vi "XML Reader Start Section.vi"(6 "Default Attribute Values":variant[](array[variant]), 7 "Attribute Names":string[](array[string]), 8 "error in":errorcluster, 10 "Element Name":string, 11 "XML Reader In":T1) -> (0 "error out":errorcluster, 1 "Attribute Values":variant[](array[variant]), 2 "Found?":bool, 3 "XML Reader Out":T1)   [LabVIEW 2018, in "Pathloss XML Reader.lvlib"]
uses:
  Pathloss XML Reader.lvlib
  Controls/XML Reader Data Ref.ctl
  Controls/XML Reader Data.ctl
  <vilib>/Utility/VariantDataType/VariantType.lvlib
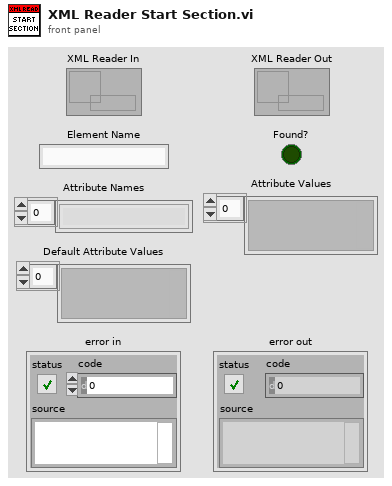
[diagram p1: front panel]
types:
  T1 = typedef "Pathloss XML Reader.lvlib/XML Reader Data Ref.ctl" = refnum<data-value>
  T2 = typedef "Pathloss XML Reader.lvlib/XML Reader Data.ctl" = cluster{"Remaining XML":string, "Section Name Stack":string[], "Section Stack":string[]}
  T3 = typedef "VariantType.lvlib/Type.ctl" = enum8{"Invalid Type", "Void", "I8", "I16", "I32", "I64", "U8", "U16", "U32", "U64", "Single Float", "Double Float", "Extended Float", "Single Complex", "Double Complex", "Extended Complex", "Enum U8", "Enum U16", "Enum U32", "Enum U64", "Single Float With Unit", "Double Float With Unit", "Extended Float With Unit", "Single Complex with Unit", "Double Complex with Unit", "Extended Complex with Unit", "Boolean", "String", "Path", "Picture", "Tag", "Array", "Cluster", "Variant", "LV Variant", "Waveform", "Timestamp", "Digital Waveform", "Digital Data", "ExpressData", "Refnum", "External Data", "VI", "Poly VI", "LabVIEW Class Instance", "Fixed Point"}
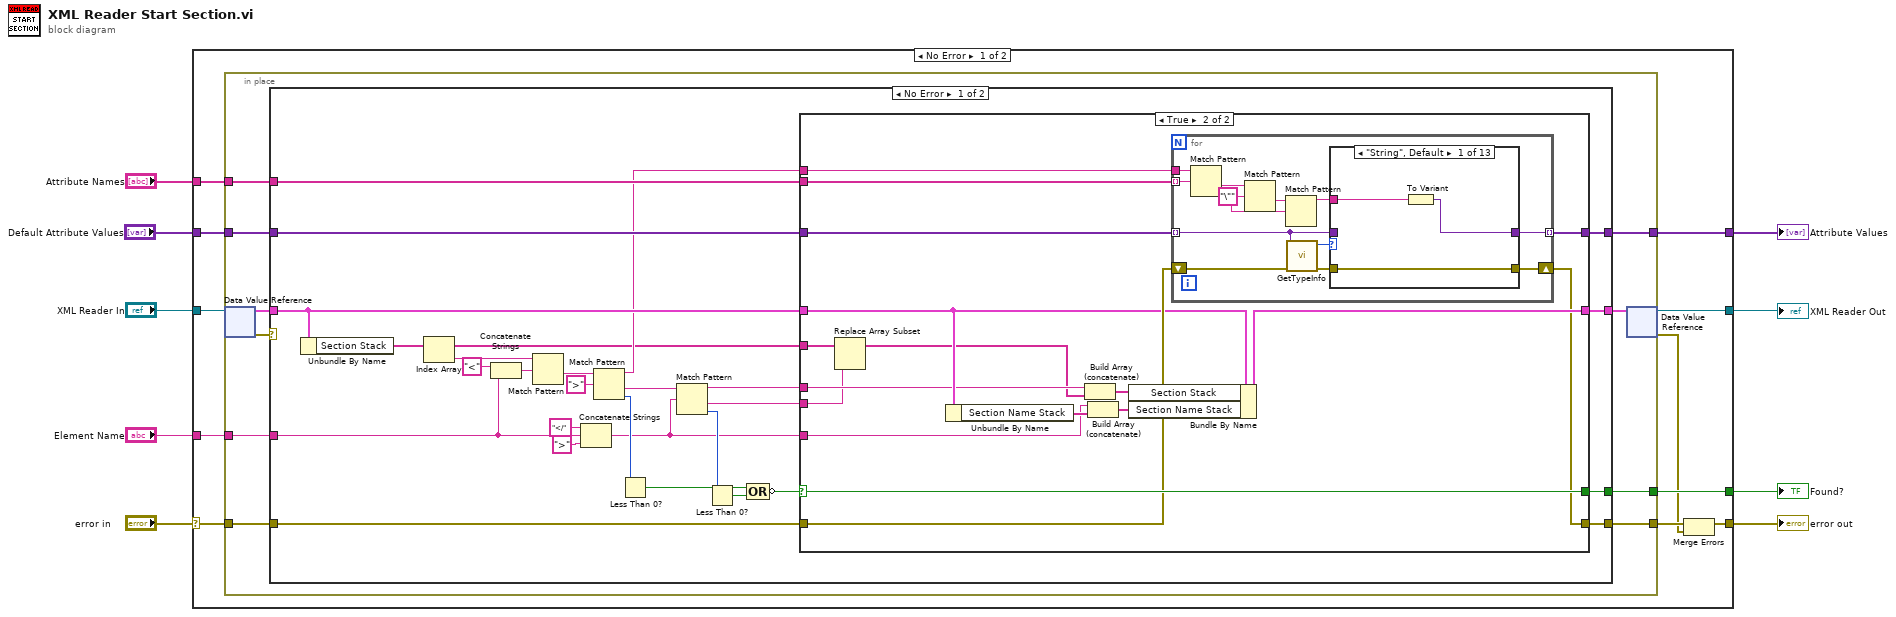
[diagram p0: block diagram]
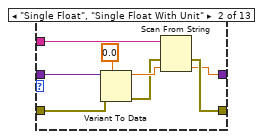
[diagram p3: hidden frame]
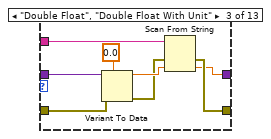
[diagram p4: hidden frame]
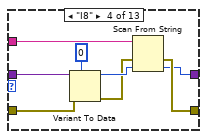
[diagram p5: hidden frame]
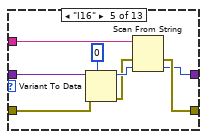
[diagram p6: hidden frame]
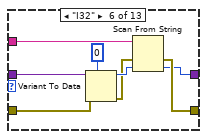
[diagram p7: hidden frame]
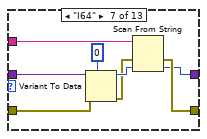
[diagram p8: hidden frame]
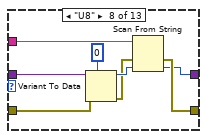
[diagram p9: hidden frame]
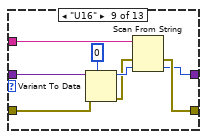
[diagram p10: hidden frame]
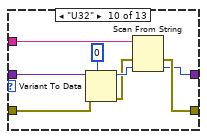
[diagram p11: hidden frame]
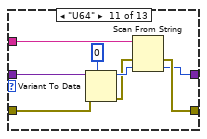
[diagram p12: hidden frame]
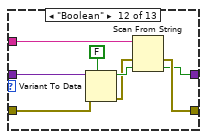
[diagram p13: hidden frame]
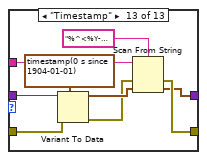
[diagram p14: hidden frame]
diagram:
  n1 = case shown="No Error" "error in" {
    selector: "error in" -> [w18 w195]
    tunnel: [w11 w195] -> w8
    tunnel: [w19 w196] -> w7
    tunnel: "XML Reader In" -> [w20 w196]
    tunnel: "Element Name" -> [w16 _]
    tunnel: "Attribute Names" -> [w15 _]
    tunnel: "Default Attribute Values" -> [w14 w194]
    tunnel: [w13 _] -> w1
    tunnel: [w12 w194] -> w2
    frame No Error {
      n2 = in-place {
        in-place-border: w18 -> [w27]
        in-place-border: [w26] -> w17
        in-place-border: w16 -> [w25]
        in-place-border: w15 -> [w24]
        in-place-border: w14 -> [w23]
        in-place-border: [w22] -> w13
        in-place-border: [w21] -> w12
        n3 = in-place-dvr #1(w20) -> (w29:T2, w30:errorcluster)
        n4 = case shown="No Error" w30 {
          selector: w30 -> [_ w192]
          tunnel: w29 -> [w48 w193]
          tunnel: [w47 w193] -> w28
          tunnel: w27 -> [w50 _]
          tunnel: [w49 w192] -> w26
          tunnel: w25 -> [w35 _]
          tunnel: w24 -> [w44 _]
          tunnel: w23 -> [w45 w191]
          tunnel: [w46 _] -> w22
          tunnel: [w43 w191] -> w21
          frame No Error {
            n5 = Unbundle By Name(w48) -> ("Section Stack"=w39:string[])
            n6 = Index Array(array=w39) -> (element=w40:string)  [unwired: 1 in]
            n7 = Concatenate Strings("<" ("string"), w35) -> (w56:string)
            n8 = Match Pattern(string=w40, regular expression=w56) -> (after substring=w55:string)  [unwired: 1 in, 3 out]
            n9 = Concatenate Strings("</" ("string"), w35, ">" ("string")) -> (w32:string)
            n10 = Match Pattern(string=w55, regular expression=">") -> (before substring=w42:string, after substring=w36:string, offset past match=w41:i32)  [unwired: 1 in, 1 out]
            n11 = Less Than 0?(x=w41) -> (x < 0?=w53:bool)
            n12 = Match Pattern(string=w36, regular expression=w32) -> (before substring=w33:string, after substring=w31:string, offset past match=w34:i32)  [unwired: 1 in, 1 out]
            n13 = Less Than 0?(x=w34) -> (x < 0?=w52:bool)
            n14 = Compound Arithmetic op=OR(w53, w52) -> (invert w51:bool)
            n15 = case shown="True" w51 {
              selector: w51 -> [w59 w77]
              tunnel: w50 -> [w60 w71]
              tunnel: [w60 w73] -> w49
              tunnel: w48 -> [w61 w70]
              tunnel: [w61 w78] -> w47
              tunnel: w42 -> [_ w75]
              tunnel: [w59 w77] -> w46
              tunnel: w45 -> [w58 w74]
              tunnel: w44 -> [_ w76]
              tunnel: [w58 w72] -> w43
              tunnel: w32 -> [_ w68]
              tunnel: w39 -> [_ w64]
              tunnel: w33 -> [_ w65]
              tunnel: w31 -> [_ w62]
              frame False {
              }
              frame True {
                n16 = Replace Array Subset(array=w64, new element=w62) -> (w63:string[])  [unwired: 1 in]
                n17 = Unbundle By Name(w70) -> ("Section Name Stack"=w69:string[])
                n18 = Build Array (concatenate)(w65, w63) -> (w66:string[])
                n19 = Build Array (concatenate)(w68, w69) -> (w67:string[])
                n20 = Bundle By Name(cluster=w70, "Section Stack"=w66, "Section Name Stack"=w67) -> (w78:T2)
                n21 = for {
                  tunnel: w75 -> [w90]
                  tunnel: w76 -> [w89] mode=indexing
                  tunnel: w74 -> [w82] mode=indexing
                  shift-right: [w80] -> w73
                  shift-left: w71 -> [w85]
                  tunnel: [w79] -> w72 mode=indexing
                  w86 = "\"" ("regular expression")
                  n22 = Match Pattern(string=w90, regular expression=w89) -> (after substring=w88:string)  [unwired: 1 in, 3 out]
                  n23 = Match Pattern(string=w88, regular expression=w86) -> (after substring=w87:string)  [unwired: 1 in, 3 out]
                  n24 = Match Pattern(string=w87, regular expression=w86) -> (before substring=w83:string)  [unwired: 1 in, 3 out]
                  n25 = call <vilib>:"GetTypeInfo.vi"("error in (no error)"=w85, "Variant"=w82) -> ("error out"=w81:errorcluster, "Type Enum"=w84:T3)  [unwired: 5 in, 3 out]
                  n26 = case shown="\"String\", Default" w84 {
                    tunnel: w83 -> [w92 w101 w109 w117 w125 w133 w141 w149 w157 w165 w173 w181 w190]
                    tunnel: w82 -> [_ w100 w108 w116 w124 w132 w140 w148 w156 w164 w172 w180 w189]
                    tunnel: w81 -> [w93 w99 w107 w115 w123 w131 w139 w147 w155 w163 w171 w179 w188]
                    tunnel: [w93 w96 w104 w112 w120 w128 w136 w144 w152 w160 w168 w176 w185] -> w80
                    tunnel: [w91 w94 w102 w110 w118 w126 w134 w142 w150 w158 w166 w174 w183] -> w79
                    frame "String", Default {
                      n27 = To Variant(anything=w92) -> (Variant=w91:variant)
                    }
                    frame "Single Float", "Single Float With Unit" {
                      n28 = Variant To Data(error in=w99, type=sgl 0.0, Variant=w100) -> (data=w98:sgl, error out=w97:errorcluster)
                      n29 = Scan From String(input string=w101, error in=w97, default 1=w98) -> (error out=w96:errorcluster, output 1=w94:sgl)  [unwired: 2 in, 2 out]
                    }
                    frame "Double Float", "Double Float With Unit" {
                      n30 = Variant To Data(error in=w107, type=0.0, Variant=w108) -> (data=w106:dbl, error out=w105:errorcluster)
                      n31 = Scan From String(input string=w109, error in=w105, default 1=w106) -> (error out=w104:errorcluster, output 1=w102:dbl)  [unwired: 2 in, 2 out]
                    }
                    frame "I8" {
                      n32 = Variant To Data(error in=w115, type=i8 0, Variant=w116) -> (data=w114:i8, error out=w113:errorcluster)
                      n33 = Scan From String(input string=w117, error in=w113, default 1=w114) -> (error out=w112:errorcluster, output 1=w110:i8)  [unwired: 2 in, 2 out]
                    }
                    frame "I16" {
                      n34 = Variant To Data(error in=w123, type=i16 0, Variant=w124) -> (data=w122:i16, error out=w121:errorcluster)
                      n35 = Scan From String(input string=w125, error in=w121, default 1=w122) -> (error out=w120:errorcluster, output 1=w118:i16)  [unwired: 2 in, 2 out]
                    }
                    frame "I32" {
                      n36 = Variant To Data(error in=w131, type=0, Variant=w132) -> (data=w130:i32, error out=w129:errorcluster)
                      n37 = Scan From String(input string=w133, error in=w129, default 1=w130) -> (error out=w128:errorcluster, output 1=w126:i32)  [unwired: 2 in, 2 out]
                    }
                    frame "I64" {
                      n38 = Variant To Data(error in=w139, type=i64 0, Variant=w140) -> (data=w138:i64, error out=w137:errorcluster)
                      n39 = Scan From String(input string=w141, error in=w137, default 1=w138) -> (error out=w136:errorcluster, output 1=w134:i64)  [unwired: 2 in, 2 out]
                    }
                    frame "U8" {
                      n40 = Variant To Data(error in=w147, type=u8 0, Variant=w148) -> (data=w146:u8, error out=w145:errorcluster)
                      n41 = Scan From String(input string=w149, error in=w145, default 1=w146) -> (error out=w144:errorcluster, output 1=w142:u8)  [unwired: 2 in, 2 out]
                    }
                    frame "U16" {
                      n42 = Variant To Data(error in=w155, type=u16 0, Variant=w156) -> (data=w154:u16, error out=w153:errorcluster)
                      n43 = Scan From String(input string=w157, error in=w153, default 1=w154) -> (error out=w152:errorcluster, output 1=w150:u16)  [unwired: 2 in, 2 out]
                    }
                    frame "U32" {
                      n44 = Variant To Data(error in=w163, type=u32 0, Variant=w164) -> (data=w162:u32, error out=w161:errorcluster)
                      n45 = Scan From String(input string=w165, error in=w161, default 1=w162) -> (error out=w160:errorcluster, output 1=w158:u32)  [unwired: 2 in, 2 out]
                    }
                    frame "U64" {
                      n46 = Variant To Data(error in=w171, type=u64 0, Variant=w172) -> (data=w170:u64, error out=w169:errorcluster)
                      n47 = Scan From String(input string=w173, error in=w169, default 1=w170) -> (error out=w168:errorcluster, output 1=w166:u64)  [unwired: 2 in, 2 out]
                    }
                    frame "Boolean" {
                      n48 = Variant To Data(error in=w179, type=FALSE, Variant=w180) -> (data=w178:bool, error out=w177:errorcluster)
                      n49 = Scan From String(input string=w181, error in=w177, default 1=w178) -> (error out=w176:errorcluster, output 1=w174:bool)  [unwired: 2 in, 2 out]
                    }
                    frame "Timestamp" {
                      n50 = Variant To Data(error in=w188, type=timestamp(0 s since 1904-01-01), Variant=w189) -> (data=w187:timestamp, error out=w186:errorcluster)
                      n51 = Scan From String(format string="%^<%Y-%m-%dT%H:%M:%S%7u%z>T" ("regular expression"), input string=w190, error in=w186, default 1=w187) -> (error out=w185:errorcluster, output 1=w183:timestamp)  [unwired: 1 in, 2 out]
                    }
                  }
                }
              }
            }
          }
          frame Error {
          }
        }
        n52 = in-place-dvr #1(w28) -> (w19:T1, w10:errorcluster)
      }
      n53 = Merge Errors(w17, w10) -> (w11:errorcluster)
    }
    frame Error {
    }
  }
  "error out" <- w8
  "XML Reader Out" <- w7
  "Attribute Values" <- w2
  "Found?" <- w1
